vi "Read Controller.vi"(8 "error in (no error)":errorcluster, 11 "View in":refnum<class "View.lvclass">) -> (0 "error out":errorcluster, 2 "Container.lvlib:Controller.lvclass":refnum<class "Controller.lvclass">, 3 "View out":refnum<class "View.lvclass">)   [LabVIEW 2020, in "Container.lvlib" / "View.lvclass"]
uses:
  View.lvclass
  View.lvclass/View.ctl
  C:/Users/N Tan/Documents/2-Prototypes/MVC/Container/View/View.lvclass
  C:/Users/N Tan/Documents/2-Prototypes/MVC/Container/InterfaceView/InterfaceView.lvclass
  Controller/Controller.lvclass
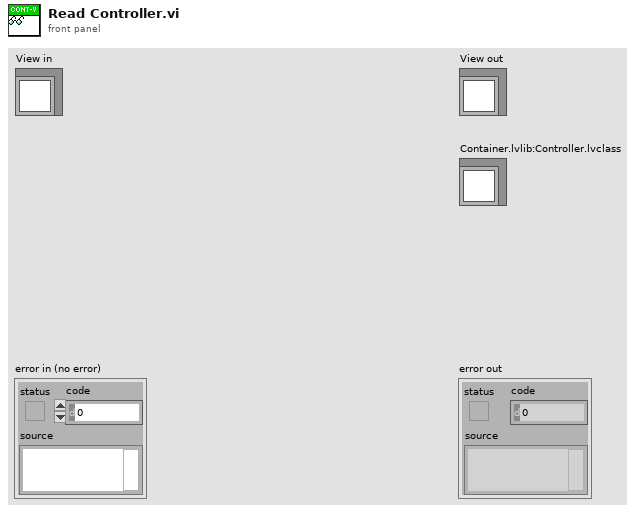
[diagram p1: front panel]
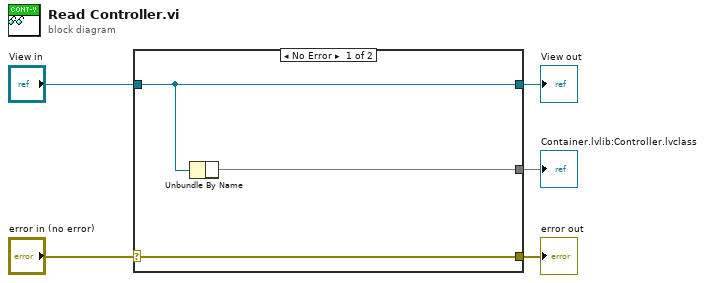
[diagram p0: block diagram]
diagram:
  n1 = case shown="No Error" "error in (no error)" {
    selector: "error in (no error)" -> [w8 w9]
    tunnel: [w8 w9] -> w4
    tunnel: [w7 w10] -> w2
    tunnel: "View in" -> [w7 w10]
    tunnel: [w6 _] -> w1
    frame No Error {
      n2 = Unbundle By Name(w7) -> (w6)
    }
    frame Error {
    }
  }
  "error out" <- w4
  "View out" <- w2
  "Container.lvlib:Controller.lvclass" <- w1
